vi "PH_Stepmotor_BaseClass.Axis Settings to Data String.vi"(1 "Axis Settings":T1) -> (0 "Data String":string)   [LabVIEW 2014, in "PH_Stepmotor_BaseClass.lvlib"]
doc: "This VI converts a specific cluster \"Axis Settings\" to a string; the cluster arguments are seperated by \"::\"."
uses:
  PH_Stepmotor_BaseClass.lvlib
  PH_Stepmotor_BaseClass.Axis Settings.ctl
  PH_Stepmotor_BaseClass.Motor Type.ctl
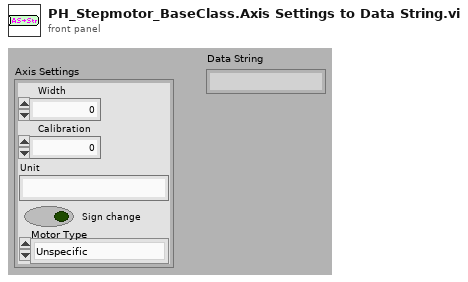
[diagram p1: front panel]
types:
  T1 = typedef "PH_Stepmotor_BaseClass.lvlib/PH_Stepmotor_BaseClass.Axis Settings.ctl" = cluster{"Sign change":bool, "Width":dbl, "Calibration":dbl, "Unit":string, "Motor Type":T2, "Unit Width":string, "Unit CF":string}
  T2 = typedef "PH_Stepmotor_BaseClass.lvlib/PH_Stepmotor_BaseClass.Motor Type.ctl" = enum16{"Unspecific", "OWIS 49.120.2633", "OWIS 49.060.1033", "OWIS 43.040.2558", "Diamond Motion 2200 series", "OWIS 49.120.266B.MV6", "Calorimeter", "Linear Stage 1", "MICOS VT-80", "MICOS VT-80 S", "Standa Rotstage nt0.95A", "PUF RA 320.200", "PUF RA 800.200", "PUF RA 800.400", "PUF RA 400.50", "1324.nn.800.50", "1324.n9c.800.50", "1324.nn.320.200", "1324.nn.400.200", "1324.nn.800.200", "1324.nn.400.50", "1324.8c9c.800.50", "1324.8c9c.400.200"}
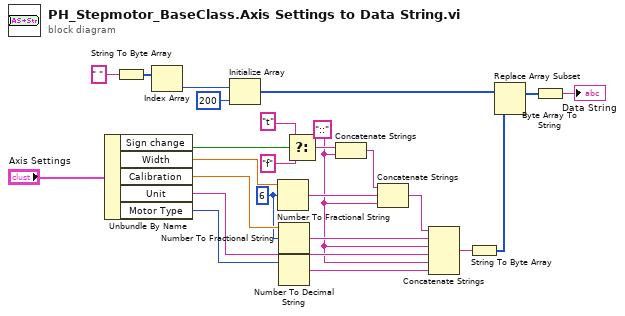
[diagram p0: block diagram]
diagram:
  w17 = i16 6 ("width (-)")
  w3 = "::"
  n1 = Unbundle By Name("Axis Settings") -> ("Sign change"=w16:bool, "Width"=w23:dbl, "Calibration"=w22:dbl, "Unit"=w18:string, "Motor Type"=w2:T2)
  n2 = String To Byte Array(string=" ") -> (unsigned byte array=w10:u8[])
  n3 = Index Array(array=w10) -> (element=w9:u8)  [unwired: 1 in]
  n4 = Initialize Array(w9, 200 ("dimension size")) -> (w6:u8[])
  n5 = Number To Fractional String(number=w23, width (-)=w17) -> (F-format string=w21:string)  [unwired: 2 in]
  n6 = Number To Fractional String(number=w22, width (-)=w17) -> (F-format string=w19:string)  [unwired: 2 in]
  n7 = Number To Decimal String(number=w2) -> (decimal integer string=w1:string)  [unwired: 1 in]
  n8 = Select(t="t", s=w16, f="f") -> (s? t:f=w13:string)
  n9 = Concatenate Strings(w13, w3) -> (w24:string)
  n10 = Concatenate Strings(w24, w21, w3) -> (w20:string)
  n11 = Concatenate Strings(w20, w19, w3, w18, w3, w1) -> (w8:string)
  n12 = String To Byte Array(string=w8) -> (unsigned byte array=w7:u8[])
  n13 = Replace Array Subset(array=w6, new element=w7) -> (w5:u8[])  [unwired: 1 in]
  n14 = Byte Array To String(unsigned byte array=w5) -> (string=→"Data String":string)
